vi "Condiciones_And_Greater_String_observaciones.vi"() -> ()   [LabVIEW 2013]
panel:
  out "Velocidad":i32(knob) scale=0.0..180.0
  out "Alarma":string
  out "Observacion":string
  out "Alarma":bool
  out "Temperatura":dbl(slide) scale=0.0..100.0
  # "Generar la temperatura entre 1-100 y la velocidad entre 1-180 cuando la velocidad sea \nmayor a 100 debemos de escribir velocidad ALTA y cuando la temperatura sea mayor a 80\ny la velocidad mayor a 120, se debe encender la alarma."
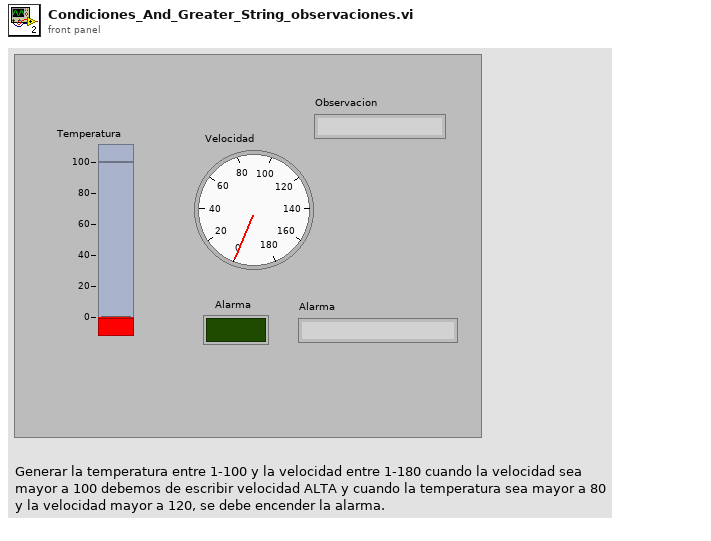
[diagram p1: front panel]
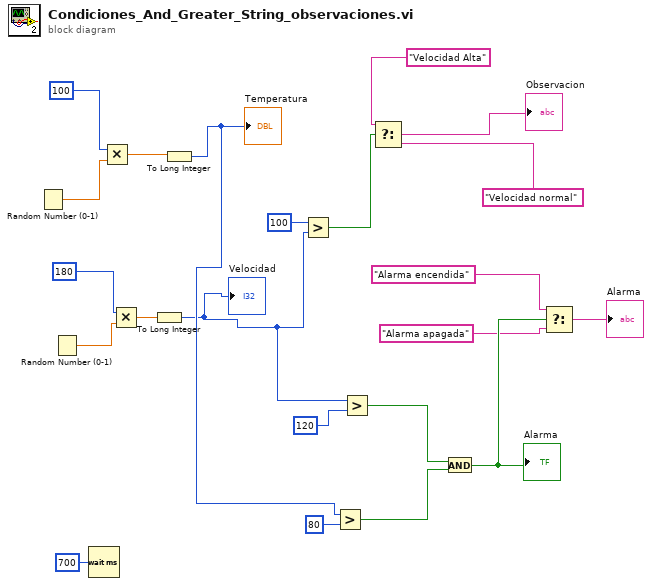
[diagram p0: block diagram]
diagram:
  n1 = Random Number (0-1)() -> (number: 0 to 1=w21:dbl)
  n2 = Random Number (0-1)() -> (number: 0 to 1=w20:dbl)
  n3 = Wait (ms)(milliseconds to wait=u32 700) -> ()  [unwired: 1 out]
  n4 = Multiply(x=100, y=w21) -> (x*y=w18:dbl)
  n5 = Multiply(x=180, y=w20) -> (x*y=w17:dbl)
  n6 = To Long Integer(number=w17) -> (32bit integer=w2:i32)
  "Velocidad" <- w2
  n7 = To Long Integer(number=w18) -> (32bit integer=w10:i32)
  "Temperatura" <- w10
  n8 = Greater?(x=100, y=w2) -> (0:w13:bool)
  n9 = Greater?(x=w10, y=80) -> (0:w7:bool)
  n10 = Greater?(x=w2, y=120) -> (0:w8:bool)
  n11 = Select(t="Velocidad Alta", s=w13, f="Velocidad normal") -> (s? t:f=→"Observacion":string)
  n12 = And(x=w8, y=w7) -> (x .and. y?=w6:bool)
  "Alarma" <- w6
  n13 = Select(t="Alarma encendida", s=w6, f="Alarma apagada") -> (s? t:f=→"Alarma":string)
